vi "PC_ParallelCaller.vi"(8 "error in (no error)":errorcluster caption="Error In (no error)", 11 "StepParameter":T2[](array[typedef])) -> (0 "error out":errorcluster, 3 "StepParameterOut":T1[](array[typedef]))   [LabVIEW 2010]
uses:
  Ctls/PC_DynCallVIParameter.ctl
  Ctls/PC_DynCallVIOutputParameter.ctl
  <vilib>/Pansino Software/LabVIEW Architecture/PSARC_Queue Management.llb/PSARC_Queue Create_Single.vi
  <vilib>/Pansino Software/LabVIEW Architecture/PSARC_Queue Management.llb/PSARC_Queue Remove Element.vi
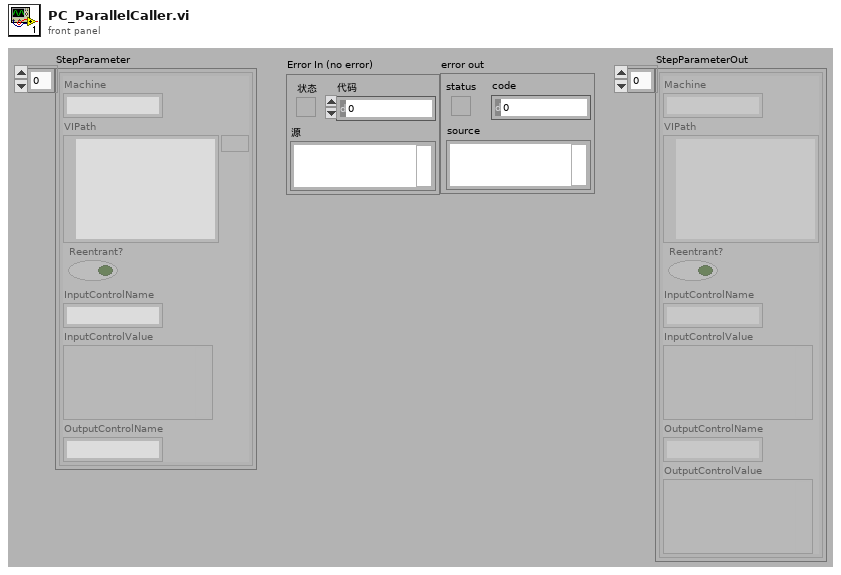
[diagram p1: front panel]
types:
  T1 = typedef "PC_DynCallVIOutputParameter.ctl" = cluster{"Machine":string, "VIPath":path, "Reentrant?":bool, "InputControlName":string, "InputControlValue":variant, "OutputControlName":string, "OutputControlValue":variant}
  T2 = typedef "PC_DynCallVIParameter.ctl" = cluster{"Machine":string, "VIPath":path, "Reentrant?":bool, "InputControlName":string, "InputControlValue":variant, "OutputControlName":string}
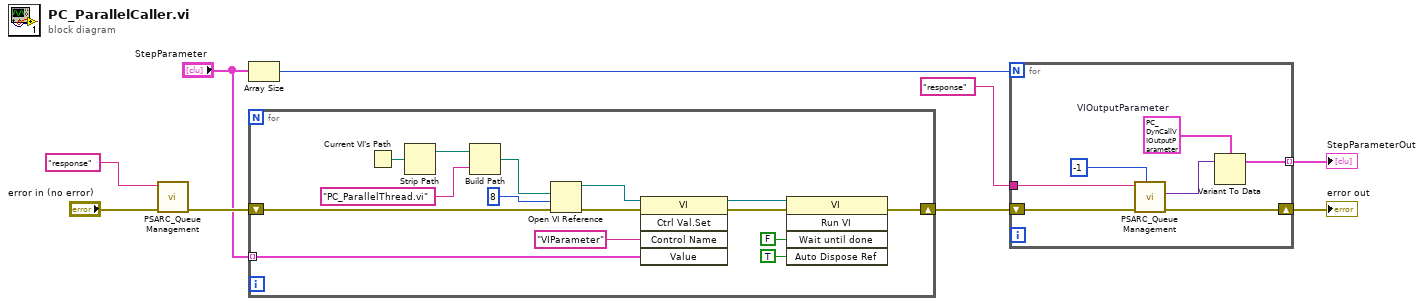
[diagram p0: block diagram]
diagram:
  n1 = call-poly <vilib>:"PSARC_Queue Management.vi"("error in (no error)"="error in (no error)", "Queue Name"="response") -> ("error out"=w9:errorcluster)  [unwired: 8 in, 1 out]
  n2 = Array Size(array="StepParameter") -> (size(s)=w6:i32)
  n3 = for {
    tunnel: "StepParameter" -> [w16] mode=indexing
    shift-right: [w14] -> w8
    shift-left: w9 -> [w15]
    n4 = Current VI's Path() -> (path=w11:path)
    n5 = Strip Path(path=w11) -> (stripped path=w12:path)  [unwired: 1 out]
    n6 = Build Path(base path=w12, name or relative path="PC_ParallelThread.vi") -> (appended path=w10:path)
    n7 = Open VI Reference(vi path=w10, options=8, error in (no error)=w15) -> (vi reference=w22:refnum<vi>, error out=w21:errorcluster)  [unwired: 3 in]
    n8 = invoke class="VI" method="Ctrl Val.Set"(reference=w22, error in=w21, "Control Name"="VIParameter", "Value"=w16) -> (reference out=w19:refnum<vi>, error out=w20:errorcluster)  [unwired: 1 in, 3 out]
    n9 = invoke class="VI" method="Run VI"(reference=w19, error in=w20, "Wait until done"=FALSE ("Wait Until Done"), "Auto Dispose Ref"=TRUE ("Auto Dispose Reference")) -> (error out=w14:errorcluster)  [unwired: 1 in, 4 out]
  }
  n10 = for {
    N: w6 -> [_]
    tunnel: "response" ("Queue Name") -> [w28]
    tunnel: [w25] -> w4 mode=indexing
    shift-right: [w30] -> w2
    shift-left: w8 -> [w31]
    w27 = T1 {"Machine"="192.168.120.8", "VIPath"=path "C:/ni-rt/startup/Test.vi", "Reentrant?"=FALSE, "InputControlName"="InputControl", "InputControlValue"=variant, "OutputControlName"="", "OutputControlValue"=variant}  # VIOutputParameter
    n11 = call-poly <vilib>:"PSARC_Queue Management.vi"("Time out(-1)_queue out"=-1, "error in (no error)"=w31, "Queue Name(unamed)"=w28) -> ("error out"=w30:errorcluster, "Data"=w26:variant)  [unwired: 5 in, 2 out]
    n12 = Variant To Data(Variant=w26, type=w27) -> (data=w25:T1)  [unwired: 1 in, 1 out]
  }
  "StepParameterOut" <- w4
  "error out" <- w2
